vi "Test.vi"() -> (0 "error out":errorcluster)   [LabVIEW 2022 SP3, in "PythonWrapper.lvlib"]
uses:
  PythonWrapper.lvlib
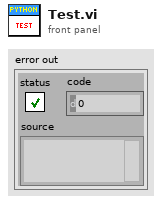
[diagram p1: front panel]
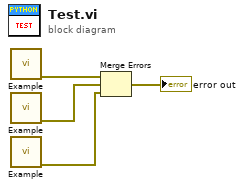
[diagram p0: block diagram]
diagram:
  n1 = call "Example.vi"() -> ("error out"=w4:errorcluster)  [unwired: 11 in]
  n2 = call "Example.vi"() -> ("error out"=w3:errorcluster)  [unwired: 11 in]
  n3 = call "Example.vi"() -> ("error out"=w2:errorcluster)  [unwired: 11 in]
  n4 = Merge Errors(w4, w3, w2) -> (→"error out":errorcluster)
